vi "Teleop.vi"(10 "Match Info":T1={"Autonomous Elapsed Seconds"=0.0, "TeleOp Elapsed Seconds"=0.0, "Disabled Elapsed Seconds"=0.0, "Visited Autonomous"=FALSE, "Visited TeleOp"=FALSE, "Visited Disabled"=FALSE, "Autonomous Settings"={"Autonomous Style"=enum."Independent", "VI Refnum"=refnum}}, 11 "Call Context":T2) -> ()   [LabVIEW 2014]
doc: "This VI is called for each TeleOp packet received from the DS where the robot is not disabled. It is often used to read from the joysticks and update I/O or to update setpoints for timed control loops. It should complete and return within 20 milliseconds or it may miss DS packets."
uses:
  <vilib>/Rock Robotics/WPI/DriverStation/WPI_DriverStationDerivedRobotMode.ctl
  <vilib>/Rock Robotics/WPI/DriverStation/WPI_DriverStationMatch Info.ctl
  Driver Names Type.ctl
  <vilib>/Rock Robotics/WPI/CAN/Jaguar/SubVIs/WPI_CANJaguar_BrakeCoastMode.ctl
  <vilib>/Rock Robotics/WPI/Solenoid/WPI_SolenoidValue.ctl
  Intake Actions.ctl
  <vilib>/Rock Robotics/WPI/Joystick/WPI_JoystickGetSetRefNum.vi
  Robot Global Data.vi
  <vilib>/addons/control/pid/pid.llb/PID Output Rate Limiter (DBL).vi
  <vilib>/Rock Robotics/WPI/RobotDrive/WPI_RobotDriveGetSetRefNum.vi
  Auto Pickup Global.vi
  <vilib>/Rock Robotics/WPI/Solenoid/WPI_SolenoidSetEnum.vi
  <vilib>/addons/control/pid/NI_PID_pid.lvlib
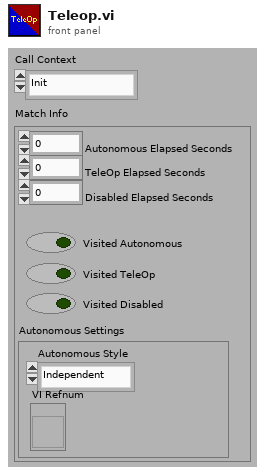
[diagram p1: front panel]
types:
  T1 = typedef "WPI_DriverStationMatch Info.ctl" = cluster{"Autonomous Elapsed Seconds":dbl, "TeleOp Elapsed Seconds":dbl, "Disabled Elapsed Seconds":dbl, "Visited Autonomous":bool, "Visited TeleOp":bool, "Visited Disabled":bool, "Autonomous Settings":cluster{"Autonomous Style":enum16{"Iterative", "Independent"}, "VI Refnum":refnum<vi>}}
  T2 = typedef "WPI_DriverStationDerivedRobotMode.ctl" = enum16{"Init", "Execute", "Stop"}
  T3 = typedef "Driver Names Type.ctl" = enum16{"Recker", "Tank"}
  T4 = typedef "WPI_JoystickDevRef.ctl" = cluster{"Device":T5}
  T5 = typedef "WPI_JoystickDeviceEnum.ctl" = enum16{"USB 0", "USB 1", "USB 2", "USB 3", "USB 4", "USB 5"}
  T6 = cluster{"Button 1":bool, "Button 2":bool, "Button 3":bool, "Button 4":bool, "Button 5":bool, "Button 6":bool, "Button 7":bool, "Button 8":bool, "Button 9":bool, "Button 10":bool, "Button 11":bool, "Button 12":bool}
  T7 = cluster{"axis 1 (x)":dbl, "axis 2 (y)":dbl, "axis 3 (throttle)":dbl, "axis 4":dbl, "axis 5":dbl, "axis 6":dbl}
  T8 = typedef "WPI_RobotDriveDevRef.ctl" = cluster{"DevStatus":errorcluster, "Motors[]":T9[], "Square Inputs":bool, "Max Output":dbl}
  T9 = typedef "WPI_MotorControlDeviceRef.ctl" = cluster{"DeviceStatus":errorcluster, "Type":enum16{"PWM", "CAN"}, "PWM":cluster{"Digital Module":T10, "PWM Channel":T11, "DeadBand":T12}, "CAN":cluster{"Device Number":u8, "Control Mode":T13, "Semaphore":T14, "Max Vout":dbl}, "Invert":bool, "TransformRef":T15, "InvTransformRef":T15}
  T10 = typedef "FPGA_TypedefDigitalModule.ctl" = enum16{"Digital Module 1", "Digital Module 2"}
  T11 = typedef "FPGA_DIOPWMChannel.ctl" = enum8{"PWM 1", "PWM 2", "PWM 3", "PWM 4", "PWM 5", "PWM 6", "PWM 7", "PWM 8", "PWM 9", "PWM 10", "Invalid"}
  T12 = typedef "WPI_PWMDeadband.ctl" = cluster{"Name":string, "maxPositivePwm":i32, "minPositivePwm":i32, "centerPwm":i32, "maxNegativePwm":i32, "minNegativePwm":i32, "angularRange":u16}
  T13 = typedef "WPI_CANJaguar_ControlMode.ctl" = enum8{"Percent VBus", "Current", "Speed", "Position", "Voltage"}
  T14 = typedef "Semaphore RefNum" = refnum<k1>
  T15 = typedef "WPI_PWMTransform_ConPane.ctl" = refnum<vi>
  T16 = typedef "WPI_CANJaguar_BrakeCoastMode.ctl" = enum8{"Jumper", "Brake", "Coast"}
  T17 = typedef "WPI_SolenoidValue.ctl" = enum16{"Off", "On", "Forward", "Reverse"}
  T18 = typedef "WPI_SolenoidDevRef.ctl" = cluster{"DevStatus":errorcluster, "Solenoid Module":T19, "Forward Solenoid Channel":T20, "Reverse Solenoid Channel":T20}
  T19 = typedef "FPGA_TypedefSolenoidModule.ctl" = enum16{"Solenoid Module 1", "Solenoid Module 2"}
  T20 = typedef "WPI_SolenoidChannel.ctl" = enum8{"Solenoid 1", "Solenoid 2", "Solenoid 3", "Solenoid 4", "Solenoid 5", "Solenoid 6", "Solenoid 7", "Solenoid 8", "Invalid"}
  T21 = typedef "Intake Actions.ctl" = enum16{"Extend", "Contain", "Motor Still", "Motor Outward", "Motor Inward", "Collect", "Pass", "Herd", "Contain Off", "Collect Delay Off", "Patea"}
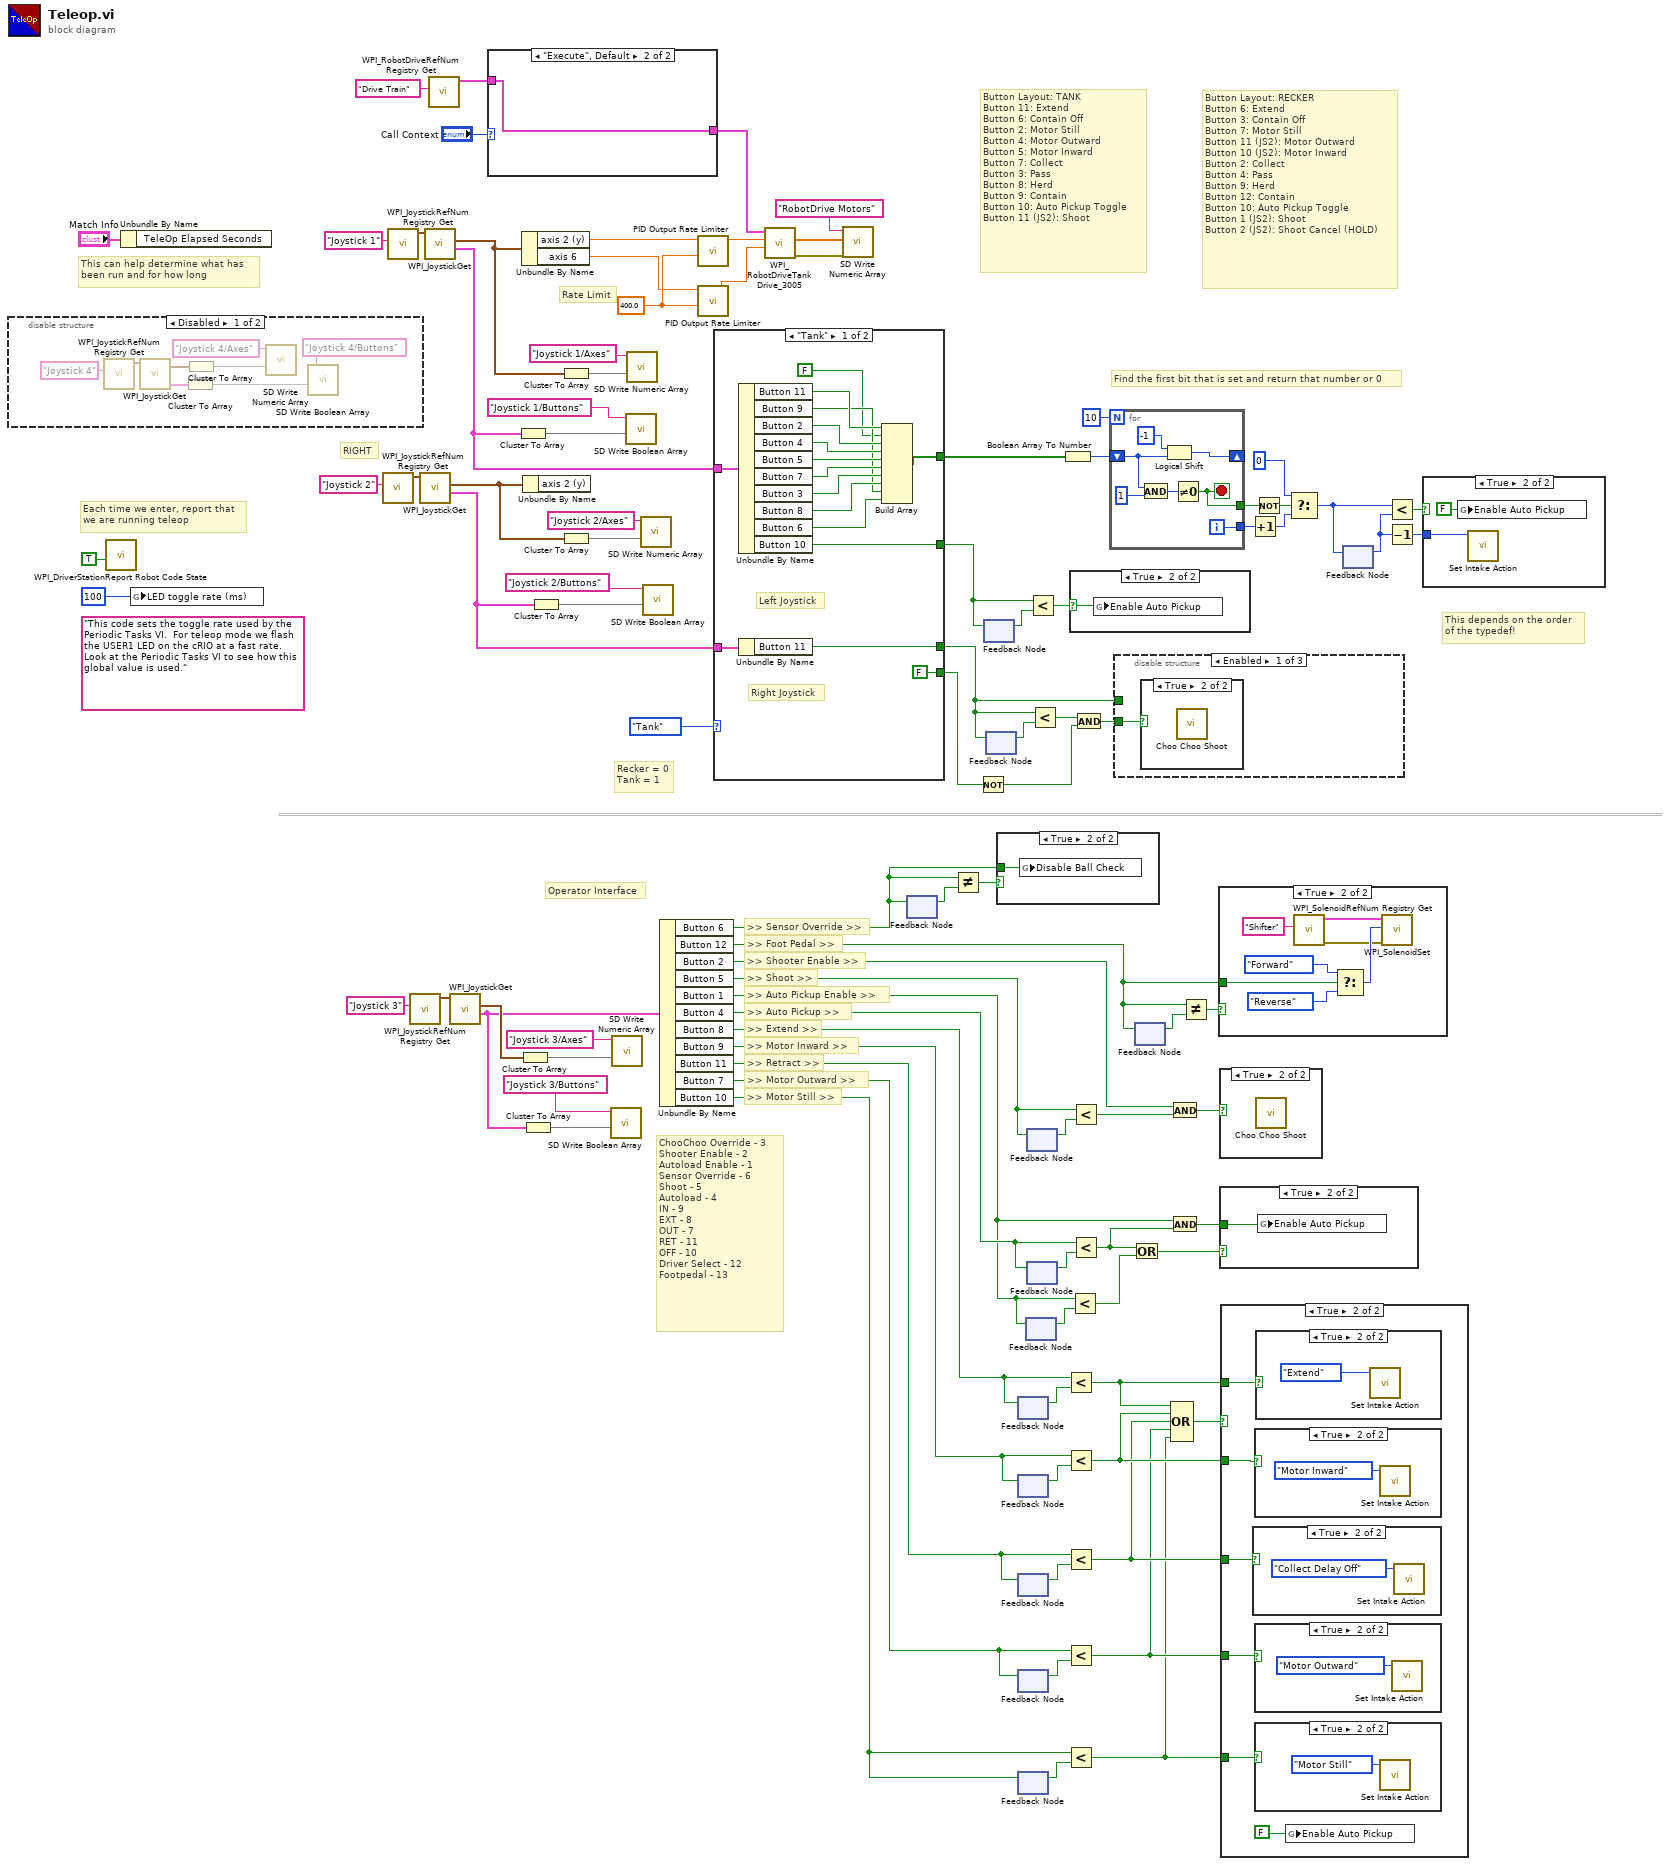
[diagram p0: block diagram]
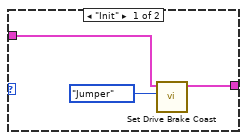
[diagram p3: hidden frame]
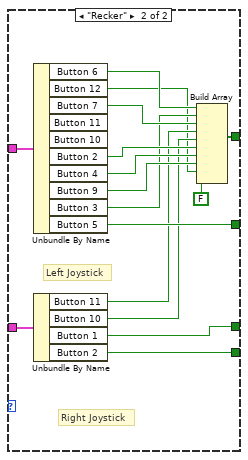
[diagram p13: hidden frame]
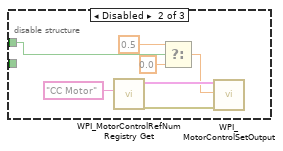
[diagram p16: hidden frame]
diagram:
  w56 = 400.0 ("output rate (EGU/min)")
  (unwired) "This code sets the toggle rate used by the Periodic Tasks VI.  For teleop mode we flash the USER1 LED on the cRIO at a fast rate.  Look at the Periodic Tasks VI to see how this global value is used."
  # "Recker = 0\nTank = 1"
  # ">> Sensor Override >>"
  # ">> Motor Still >>"
  # ">> Motor Outward >>"
  # ">> Retract >>"
  # ">> Motor Inward >>"
  # ">> Extend >>"
  # ">> Auto Pickup Enable >>"
  # ">> Auto Pickup >>"
  # ">> Shoot >>"
  # ">> Shooter Enable >>"
  # ">> Foot Pedal >>"
  # "Operator Interface"
  # "ChooChoo Override - 3\nShooter Enable - 2\nAutoload Enable - 1\nSensor Override - 6\nShoot - 5\nAutoload - 4\nIN - 9\nEXT - 8\nOUT - 7\nRET - 11\nOFF - 10\nDriver Select - 12\nFootpedal - 13"
  # "Button Layout: TANK\nButton 11: Extend\nButton 6: Contain Off\nButton 2: Motor Still\nButton 4: Motor Outward\nButton 5: Motor Inward\nButton 7: Collect\nButton 3: Pass\nButton 8: Herd\nButton 9: Contain\nButton 10: Auto Pickup Toggle\nButton 11 (JS2): Shoot"
  # "Rate Limit"
  # "RIGHT"
  # "This depends on the order\nof the typedef!"
  # "Button Layout: RECKER\nButton 6: Extend\nButton 3: Contain Off\nButton 7: Motor Still\nButton 11 (JS2): Motor Outward\nButton 10 (JS2): Motor Inward\nButton 2: Collect\nButton 4: Pass\nButton 9: Herd\nButton 12: Contain\nButton 10: Auto Pickup Toggle\nButton 1 (JS2): Shoot\nButton 2 (JS2): Shoot Cancel (HOLD)"
  # "Find the first bit that is set and return that number or 0"
  # "Each time we enter, report that\nwe are running teleop"
  # "This can help determine what has\nbeen run and for how long"
  n1 = disable-structure shown="Disabled" {
    frame Disabled {
      n2 = call <vilib>:"WPI_JoystickRefNum Registry Get.vi"("refnum name"="Joystick 4") -> ("JoystickDevRef"=w100:T4)  [unwired: 1 in, 9 out]
      n3 = call <vilib>:"WPI_JoystickGet.vi"("JoystickDevRef"=w100) -> ("Buttons"=w97:T6, "Axes"=w98:T7)  [unwired: 1 in, 4 out]
      n4 = Cluster To Array(cluster=w97) -> (array=w101:bool[])
      n5 = Cluster To Array(cluster=w98) -> (array=w103:dbl[])
      n6 = call <vilib>:"SD Write Numeric Array.vi"("Numeric Array"=w103, "Name"="Joystick 4/Axes") -> ()  [unwired: 8 in, 2 out]
      n7 = call <vilib>:"SD Write Boolean Array.vi"("Boolean Array"=w101, "Name"="Joystick 4/Buttons") -> ()  [unwired: 8 in, 2 out]
    }
    frame Enabled {
    }
  }
  n8 = call <vilib>:"WPI_DriverStationReport Robot Code State.vi"("TeleOp"=TRUE ("Autonomous")) -> ()  [unwired: 10 in, 1 out]
  n9 = Unbundle By Name("Match Info") -> ()  [unwired: 1 out]
  n10 = global write "Robot Global Data.vi" "LED toggle rate (ms)"(u32 100 ("LED ms toggle rate")) -> ()
  n11 = call <vilib>:"WPI_JoystickRefNum Registry Get.vi"("refnum name"="Joystick 2") -> ("JoystickDevRef"=w93:T4)  [unwired: 1 in, 9 out]
  n12 = call <vilib>:"WPI_JoystickRefNum Registry Get.vi"("refnum name"="Joystick 1") -> ("JoystickDevRef"=w80:T4)  [unwired: 1 in, 9 out]
  n13 = call <vilib>:"WPI_JoystickRefNum Registry Get.vi"("refnum name"="Joystick 3") -> ("JoystickDevRef"=w14:T4)  [unwired: 1 in, 9 out]
  n14 = call <vilib>:"WPI_JoystickGet.vi"("JoystickDevRef"=w93) -> ("Buttons"=w62:T6, "Axes"=w76:T7)  [unwired: 1 in, 4 out]
  n15 = call <vilib>:"WPI_JoystickGet.vi"("JoystickDevRef"=w80) -> ("Buttons"=w60:T6, "Axes"=w78:T7)  [unwired: 1 in, 4 out]
  n16 = call <vilib>:"WPI_RobotDriveRefNum Registry Get.vi"("refnum name"="Drive Train") -> ("RobotDriveDevRef"=w6:T8)  [unwired: 1 in, 9 out]
  n17 = call <vilib>:"WPI_JoystickGet.vi"("JoystickDevRef"=w14) -> ("Buttons"=w12:T6, "Axes"=w19:T7)  [unwired: 1 in, 4 out]
  n18 = case shown="\"Execute\", Default" "Call Context" {
    tunnel: w6 -> [w106 w108]
    tunnel: [w105 w108] -> w5
    frame "Init" {
      n19 = call "Set Drive Brake Coast.vi"("Brake / Coast Mode"=WPI_CANJaguar_BrakeCoastMode."Jumper", "RobotDriveDevRef"=w106) -> ("RobotDriveDevRef 2"=w105:T8)  [unwired: 8 in, 1 out]
    }
    frame "Execute", Default {
    }
  }
  n20 = Cluster To Array(cluster=w60) -> (array=w81:bool[])
  n21 = Cluster To Array(cluster=w19) -> (array=w17:dbl[])
  n22 = Unbundle By Name(w78) -> ("axis 2 (y)"=w58:dbl, "axis 6"=w1:dbl)
  n23 = Unbundle By Name(w76) -> ()  [unwired: 1 out]
  n24 = Cluster To Array(cluster=w12) -> (array=w15:bool[])
  n25 = Cluster To Array(cluster=w62) -> (array=w90:bool[])
  n26 = Cluster To Array(cluster=w78) -> (array=w83:dbl[])
  n27 = Cluster To Array(cluster=w76) -> (array=w88:dbl[])
  n28 = call <vilib>:"SD Write Boolean Array.vi"("Boolean Array"=w15, "Name"="Joystick 3/Buttons") -> ()  [unwired: 8 in, 2 out]
  n29 = call <vilib>:"SD Write Numeric Array.vi"("Numeric Array"=w17, "Name"="Joystick 3/Axes") -> ()  [unwired: 8 in, 2 out]
  n30 = call <vilib>:"SD Write Boolean Array.vi"("Boolean Array"=w81, "Name"="Joystick 1/Buttons") -> ()  [unwired: 8 in, 2 out]
  n31 = call <vilib>:"SD Write Numeric Array.vi"("Numeric Array"=w83, "Name"="Joystick 1/Axes") -> ()  [unwired: 8 in, 2 out]
  n32 = call <vilib>:"SD Write Numeric Array.vi"("Numeric Array"=w88, "Name"="Joystick 2/Axes") -> ()  [unwired: 8 in, 2 out]
  n33 = call <vilib>:"SD Write Boolean Array.vi"("Boolean Array"=w90, "Name"="Joystick 2/Buttons") -> ()  [unwired: 8 in, 2 out]
  n34 = Unbundle By Name(w12) -> ("Button 6"=w8:bool, "Button 12"=w45:bool, "Button 2"=w40:bool, "Button 5"=w41:bool, "Button 1"=w26:bool, "Button 4"=w37:bool, "Button 8"=w35:bool, "Button 9"=w32:bool, "Button 11"=w22:bool, "Button 7"=w20:bool, "Button 10"=w10:bool)
  n35 = call-poly <vilib>:"PID Output Rate Limiter.vi"("output rate (EGU/min)"=w56, "input (controller output)"=w58) -> ("output"=w57:dbl)  [unwired: 6 in, 1 out]
  n36 = call-poly <vilib>:"PID Output Rate Limiter.vi"("output rate (EGU/min)"=w56, "input (controller output)"=w1) -> ("output"=w59:dbl)  [unwired: 6 in, 1 out]
  n37 = case shown="\"Tank\"" Driver_Names_Type."Tank" {
    tunnel: [w118 w136] -> w75
    tunnel: w62 -> [w117 w135]
    tunnel: [w116 w129] -> w61
    tunnel: w60 -> [w115 w134]
    tunnel: [w113 w132] -> w53
    tunnel: [FALSE ("Button 2") w128] -> w50
    frame "Tank" {
      # "Left Joystick"
      # "Right Joystick"
      n38 = Unbundle By Name(w115) -> ("Button 11"=w114:bool, "Button 9"=w111:bool, "Button 2"=w124:bool, "Button 4"=w123:bool, "Button 5"=w122:bool, "Button 7"=w121:bool, "Button 3"=w120:bool, "Button 8"=w119:bool, "Button 6"=w110:bool, "Button 10"=w113:bool)
      n39 = Unbundle By Name(w117) -> ("Button 11"=w116:bool)
      n40 = Build Array(w114, FALSE ("element"), w124, w123, w122, w121, w120, w119, w111, w110) -> (w118:bool[])
    }
    frame "Recker" {
      # "Left Joystick"
      # "Right Joystick"
      n41 = Unbundle By Name(w134) -> ("Button 6"=w133:bool, "Button 12"=w126:bool, "Button 7"=w140:bool, "Button 2"=w139:bool, "Button 4"=w138:bool, "Button 9"=w137:bool, "Button 3"=w127:bool, "Button 5"=w132:bool)  [unwired: 2 out]
      n42 = Unbundle By Name(w135) -> ("Button 11"=w131:bool, "Button 10"=w130:bool, "Button 1"=w129:bool, "Button 2"=w128:bool)
      n43 = Build Array(w133, w127, w140, w131, w130, w139, w138, w137, w126, FALSE ("element")) -> (w136:bool[])
    }
  }
  n44 = call <vilib>:"WPI_RobotDriveTankDrive_3005.vi"("Right axis value"=w59, "Left axis value"=w57, "RobotDriveDevRef"=w5) -> ("error out"=w77:errorcluster, "Motor Values"=w85:dbl[])  [unwired: 6 in, 1 out]
  n45 = call <vilib>:"SD Write Numeric Array.vi"("error in"=w77, "Numeric Array"=w85, "Name"="RobotDrive Motors") -> ()  [unwired: 7 in, 2 out]
  n46 = feedback #1() -> (w4:bool)  [unwired: 1 in]
  n47 = feedback-in #1(w8) -> ()
  n48 = Not Equal?(x=w8, y=w4) -> (x != y?=w3:bool)
  n49 = Not(x=w50) -> (.not. x?=w49:bool)
  n50 = feedback #2() -> (w55:bool)  [unwired: 1 in]
  n51 = feedback-in #2(w53) -> ()
  n52 = feedback #3() -> (w63:bool)  [unwired: 1 in]
  n53 = feedback-in #3(w61) -> ()
  n54 = case shown="True" w3 {
    tunnel: w8 -> [_ w141]
    frame False {
    }
    frame True {
      n55 = global write "Robot Global Data.vi" "Disable Ball Check"(w141) -> ()
    }
  }
  n56 = feedback #4() -> (w36:bool)  [unwired: 1 in]
  n57 = feedback-in #4(w35) -> ()
  n58 = feedback #5() -> (w34:bool)  [unwired: 1 in]
  n59 = feedback-in #5(w32) -> ()
  n60 = feedback #6() -> (w33:bool)  [unwired: 1 in]
  n61 = feedback-in #6(w22) -> ()
  n62 = feedback #7() -> (w23:bool)  [unwired: 1 in]
  n63 = feedback-in #7(w20) -> ()
  n64 = feedback #8() -> (w11:bool)  [unwired: 1 in]
  n65 = feedback-in #8(w10) -> ()
  n66 = feedback #9() -> (w27:bool)  [unwired: 1 in]
  n67 = feedback-in #9(w26) -> ()
  n68 = feedback #10() -> (w44:bool)  [unwired: 1 in]
  n69 = feedback-in #10(w41) -> ()
  n70 = feedback #11() -> (w39:bool)  [unwired: 1 in]
  n71 = feedback-in #11(w37) -> ()
  n72 = Less?(x=w53, y=w55) -> (x < y?=w54:bool)
  n73 = Less?(x=w61, y=w63) -> (x < y?=w51:bool)
  n74 = Boolean Array To Number(Boolean array=w75) -> (number=w74:u32)
  n75 = Less?(x=w35, y=w36) -> (x < y?=w30:bool)
  n76 = Less?(x=w32, y=w34) -> (x < y?=w29:bool)
  n77 = Less?(x=w22, y=w33) -> (x < y?=w28:bool)
  n78 = Less?(x=w20, y=w23) -> (x < y?=w21:bool)
  n79 = Less?(x=w10, y=w11) -> (x < y?=w9:bool)
  n80 = case shown="True" w54 {
    selector: w54 -> [_ w142]
    frame False {
    }
    frame True {
      n81 = global write "Auto Pickup Global.vi" "Enable Auto Pickup"(w142) -> ()
    }
  }
  n82 = Less?(x=w26, y=w27) -> (x < y?=w25:bool)
  n83 = Less?(x=w41, y=w44) -> (x < y?=w43:bool)
  n84 = Less?(x=w37, y=w39) -> (x < y?=w2:bool)
  n85 = And(x=w51, y=w49) -> (x .and. y?=w48:bool)
  n86 = for {
    N: 10 -> [_]
    shift-right: [w145] -> _
    shift-left: w74 -> [w144]
    tunnel: [w147] -> w66
    tunnel: [w146] -> w73
    i -> [w147]
    stop <- w146 stop-if-true
    n87 = And(x=w144, y=u32 1) -> (x .and. y?=w148:u32)
    n88 = Logical Shift(y=i16 -1, x=w144) -> (x << y=w145:u32)
    n89 = Not Equal To 0?(x=w148) -> (x != 0?=w146:bool)
  }
  n90 = disable-structure shown="Enabled" {
    disable-tunnel: w48 -> [w150 _ _]
    disable-tunnel: w61 -> [_ w156 _]
    frame Enabled {
      n91 = case shown="True" w150 {
        frame False {
        }
        frame True {
          n92 = call "Choo Choo Shoot.vi"() -> ()  [unwired: 11 in, 1 out]
        }
      }
    }
    frame Disabled {
      n93 = call <vilib>:"WPI_MotorControlRefNum Registry Get.vi"("refnum name"="CC Motor") -> ("error out"=w151:errorcluster, "MotorControlDevRef"=w153:T9)  [unwired: 9 in]
      n94 = Select(t=0.5 ("Output"), s=w156, f=0.0) -> (s? t:f=w152:dbl)
      n95 = call <vilib>:"WPI_MotorControlSetOutput.vi"("error in (no error)"=w151, "Output"=w152, "MotorControlDevRef"=w153) -> ()  [unwired: 6 in, 3 out]
    }
    frame Disabled {
    }
  }
  n96 = Or(x=w2, y=w25) -> (x .or. y?=w24:bool)
  n97 = feedback #12() -> (w47:bool)  [unwired: 1 in]
  n98 = feedback-in #12(w45) -> ()
  n99 = And(x=w40, y=w43) -> (x .and. y?=w42:bool)
  n100 = And(x=w26, y=w2) -> (x .and. y?=w38:bool)
  n101 = Compound Arithmetic op=OR(w30, w29, w28, w21, w9) -> (w31:bool)
  n102 = Not Equal?(x=w45, y=w47) -> (x != y?=w46:bool)
  n103 = case shown="True" w46 {
    tunnel: w45 -> [_ w163]
    frame False {
    }
    frame True {
      n104 = call <vilib>:"WPI_SolenoidRefNum Registry Get.vi"("refnum name"="Shifter") -> ("error out"=w158:errorcluster, "SolenoidDevRef"=w159:T18)  [unwired: 9 in]
      n105 = Select(t=WPI_SolenoidValue."Forward" ("Value"), s=w163, f=WPI_SolenoidValue."Reverse" ("Value")) -> (s? t:f=w164:T17)
      n106 = call-poly <vilib>:"WPI_SolenoidSet.vi"("error in (no error)"=w158, "Value"=w164, "SolenoidDevRef"=w159) -> ()  [unwired: 7 in, 2 out]
    }
  }
  n107 = case shown="True" w42 {
    frame False {
    }
    frame True {
      n108 = call "Choo Choo Shoot.vi"() -> ()  [unwired: 11 in, 1 out]
    }
  }
  n109 = case shown="True" w24 {
    tunnel: w38 -> [_ w165]
    frame False {
    }
    frame True {
      n110 = global write "Auto Pickup Global.vi" "Enable Auto Pickup"(w165) -> ()
    }
  }
  n111 = case shown="True" w31 {
    tunnel: w30 -> [_ w170]
    tunnel: w29 -> [_ w169]
    tunnel: w28 -> [_ w168]
    tunnel: w21 -> [_ w167]
    tunnel: w9 -> [_ w166]
    frame False {
    }
    frame True {
      n112 = case shown="True" w168 {
        frame False {
        }
        frame True {
          n113 = call "Set Intake Action.vi"("Action"=Intake_Actions."Collect Delay Off") -> ()  [unwired: 10 in, 1 out]
        }
      }
      n114 = case shown="True" w169 {
        frame False {
        }
        frame True {
          n115 = call "Set Intake Action.vi"("Action"=Intake_Actions."Motor Inward") -> ()  [unwired: 10 in, 1 out]
        }
      }
      n116 = case shown="True" w167 {
        frame False {
        }
        frame True {
          n117 = call "Set Intake Action.vi"("Action"=Intake_Actions."Motor Outward") -> ()  [unwired: 10 in, 1 out]
        }
      }
      n118 = case shown="True" w166 {
        frame False {
        }
        frame True {
          n119 = call "Set Intake Action.vi"("Action"=Intake_Actions."Motor Still") -> ()  [unwired: 10 in, 1 out]
        }
      }
      n120 = case shown="True" w170 {
        frame False {
        }
        frame True {
          n121 = call "Set Intake Action.vi"("Action"=Intake_Actions."Extend") -> ()  [unwired: 10 in, 1 out]
        }
      }
      n122 = global write "Auto Pickup Global.vi" "Enable Auto Pickup"(FALSE ("Enable Auto Pickup")) -> ()
    }
  }
  n123 = Increment(x=w66) -> (x+1=w65:i32)
  n124 = Not(x=w73) -> (.not. x?=w68:bool)
  n125 = Select(t=0, s=w68, f=w65) -> (s? t:f=w69:i32)
  n126 = feedback #13() -> (w67:i32)  [unwired: 1 in]
  n127 = feedback-in #13(w69) -> ()
  n128 = Less?(x=w69, y=w67) -> (x < y?=w70:bool)
  n129 = Decrement(x=w67) -> (x-1=w64:i32)
  n130 = case shown="True" w70 {
    tunnel: w64 -> [_ w178]
    frame False {
    }
    frame True {
      n131 = global write "Auto Pickup Global.vi" "Enable Auto Pickup"(FALSE ("Enable Auto Pickup")) -> ()
      n132 = call "Set Intake Action.vi"("Action"=w178) -> ()  [unwired: 10 in, 1 out]
    }
  }
